vi "f4+g4u.vi"(9 "u":dbl, 10 "x4_":dbl, 11 "x3_":dbl) -> (3 "f4+g4u 2":dbl)   [LabVIEW 2014]
uses:
  <vilib>/Simulation/Implementation/Shared/SIMSCR Execution Mode.ctl
  <vilib>/Simulation/Scripting/Companion Diagram/SimConfigNode/SimParams.ctl
  <vilib>/Simulation/Scripting/Companion Diagram/SimConfigNode/_simSolvers.ctl
  <vilib>/Simulation/Param Hierarchy/Typedefs/SIMPH Param Control Actions.ctl
  <vilib>/Simulation/Implementation/Shared/NILVSim_ParamChanged.vi
  <vilib>/Simulation/Implementation/Shared/NILVSIM_BeginStep.vi
  <vilib>/Simulation/Implementation/Shared/NILVSim_Manager.vi
  <vilib>/Utility/error.llb/Clear Errors.vi
  <vilib>/Simulation/Implementation/Shared/NILVSim_FinalizeModel.vi
  <vilib>/Simulation/Implementation/Shared/SIM Unbundle Sim Info.vi
  <vilib>/Simulation/Implementation/Shared/SIMSH Read Queue.vi
  <vilib>/Simulation/Implementation/Shared/NILVSim_Initialize.vi
  <vilib>/Simulation/Utility/Implementation/NILVSim Get Time and IsAcceptedStep.vi
  <vilib>/Simulation/Implementation/Shared/NILVSim_GetModelError.vi
  <vilib>/Simulation/Implementation/Shared/SIM SimErrorHandler.vi
  <vilib>/Simulation/Implementation/Shared/SIM Bundle Sim Info.vi
  <vilib>/Simulation/Scripting/Companion Diagram/SimConfigNode/SimDog.xnode
  <vilib>/Simulation/Implementation/XNodeFramework/SimXNode/SimX.xnode
  <vilib>/Simulation/Implementation/Shared/NI_SIM_Implementation.lvlib
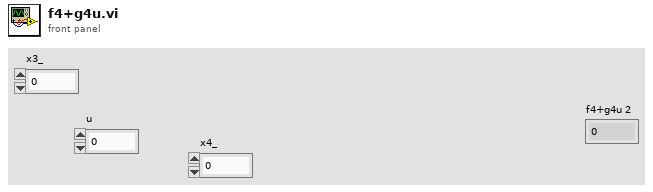
[diagram p1: front panel]
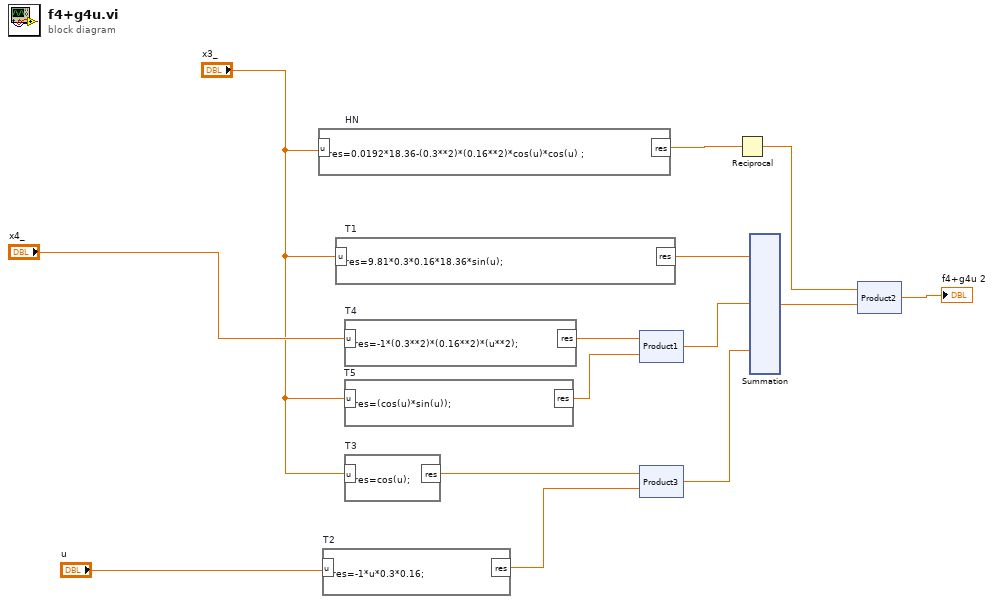
[diagram p0: block diagram]
diagram:
  n1 = formula code="res=0.0192*18.36-(0.3**2)*(0.16**2)*cos(u)*cos(u) ;" "HN"("u"="x3_") -> ("res"=w14:dbl)
  n2 = formula code="res=-1*u*0.3*0.16;" "T2"("u"="u") -> ("res"=w2:dbl)
  n3 = formula code="res=9.81*0.3*0.16*18.36*sin(u);" "T1"("u"="x3_") -> ("res"=w5:dbl)
  n4 = formula code="res=-1*(0.3**2)*(0.16**2)*(u**2);" "T4"("u"="x4_") -> ("res"=w4:dbl)
  n5 = formula code="res=(cos(u)*sin(u));" "T5"("u"="x3_") -> ("res"=w9:dbl)
  n6 = formula code="res=cos(u);" "T3"("u"="x3_") -> ("res"=w3:dbl)
  n7 = xnode "Product1"("Operand1"=w4, "Operand2"=w9) -> ("Result"=w8:dbl)
  n8 = xnode "Product3"("Operand1"=w3, "Operand2"=w2) -> ("Result"=w7:dbl)
  n9 = Reciprocal ("Math\\nFunction")(x=w14) -> (1/x=w13:dbl)
  n10 = xnode ("Summation")("Operand1"=w5, "Operand2"=w8, "Operand3"=w7) -> ("Result"=w12:dbl)
  n11 = xnode "Product2"("Operand1"=w13, "Operand2"=w12) -> ("Result"=→"f4+g4u 2":dbl)
